vi "ROI_edit_ROI_manager.vi"(3 "error in":errorcluster, 4 "XY positions":dbl[][](array[numeric]), 5 "ROI Refnum":refnum<vi>) -> (0 "error out":errorcluster)   [LabVIEW 2015]
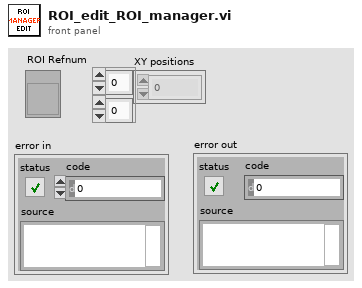
[diagram p1: front panel]
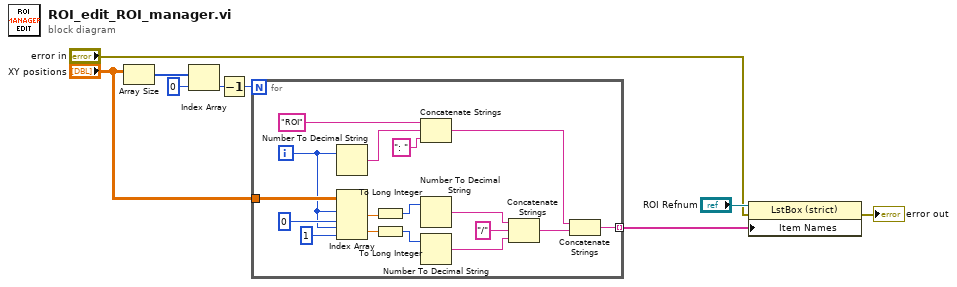
[diagram p0: block diagram]
diagram:
  n1 = Array Size(array="XY positions") -> (size(s)=w9:i32[])
  n2 = Index Array(array=w9, index=0) -> (element=w7:i32)
  n3 = Decrement(x=w7) -> (x-1=w6:i32)
  n4 = for {
    N: w6 -> [_]
    tunnel: "XY positions" -> [w26]
    tunnel: [w10] -> w4 mode=indexing
    i -> [w22]
    n5 = Number To Decimal String(number=w22) -> (decimal integer string=w21:string)  [unwired: 1 in]
    n6 = Index Array(array=w26, index (row) #1=w22, index (col) #1=0 ("disabled index (col)"), index (row) #2=w22, index (col) #2=1 ("disabled index (col)")) -> (element #1=w20:dbl, element #2=w19:dbl)
    n7 = To Long Integer(number=w20) -> (32bit integer=w18:i32)
    n8 = To Long Integer(number=w19) -> (32bit integer=w17:i32)
    n9 = Concatenate Strings("ROI", w21, ": ") -> (w12:string)
    n10 = Number To Decimal String(number=w18) -> (decimal integer string=w15:string)  [unwired: 1 in]
    n11 = Number To Decimal String(number=w17) -> (decimal integer string=w13:string)  [unwired: 1 in]
    n12 = Concatenate Strings(w15, "/" ("string"), w13) -> (w11:string)
    n13 = Concatenate Strings(w12, w11) -> (w10:string)
  }
  n14 = property class="LstBox (strict)"(reference="ROI Refnum", error in="error in", "Item Names"=w4) -> (error out=→"error out":errorcluster)  [unwired: 1 out]
